vi "XiXi-1(Add 数组移位法).vi"(10 "X[-1]":dbl, 11 "Xi":dbl[](array[numeric])) -> (3 "Yi":dbl[](array[numeric]) format="%.2f")   [LabVIEW 2012]
doc: "Calculate sums of consecutive array elements. 0th element of output is equal to x(0)+ x(-1), where x(-1) is an optional scalar input that defaults to zero."
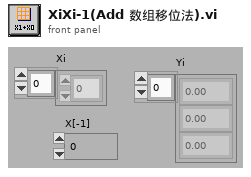
[diagram p1: front panel]
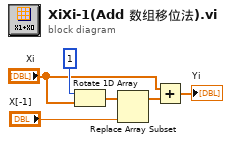
[diagram p0: block diagram]
diagram:
  n1 = Rotate 1D Array(1:"Xi", 2:1 ("n")) -> (0:w5:dbl[])
  n2 = Replace Array Subset(array=w5, new element="X[-1]") -> (w2:dbl[])  [unwired: 1 in]
  n3 = Add(x="Xi", y=w2) -> (x+y=→"Yi":dbl[])
